vi "Ctor.vi"(8 "error in (no error)":errorcluster) -> (0 "error out":errorcluster, 3 "PanelArray":refnum<class "ArrayManager.lvclass">)   [LabVIEW 2020, in "OOPanel.lvlib" / "ArrayManager.lvclass"]
uses:
  ArrayManager.lvclass
  ArrayPanel/ArrayPanel.lvclass
  UI Refs.ctl
  Events.ctl
  State Ref.ctl
  Event Regs.ctl
  ArrayManager.lvclass/ArrayManager.ctl
  Manager/Manager.lvclass
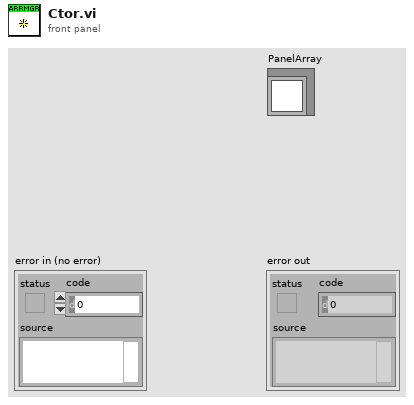
[diagram p1: front panel]
types:
  T1 = typedef "OOPanel.lvlib/ArrayManager.lvclass/Event Regs.ctl" = cluster{"Event Reg":refnum<event-registration>, "Last Update Ticks ms":u32}
  T2 = typedef "OOPanel.lvlib/ArrayManager.lvclass/State Ref.ctl" = cluster{"Running":bool, "Borders":bool, "Total Height":dbl, "Scroll Visible":bool}
  T3 = typedef "OOPanel.lvlib/ArrayManager.lvclass/Events.ctl" = cluster{"Stop":refnum<user-event>, "Update":refnum<user-event>, "Scroll":refnum<user-event>}
  T4 = typedef "OOPanel.lvlib/ArrayManager.lvclass/UI Refs.ctl" = cluster{"SubPanels":refnum<vi>[], "Scrollbar":refnum<vi>, "Panel VI":refnum<vi>, "Container":refnum<vi>}
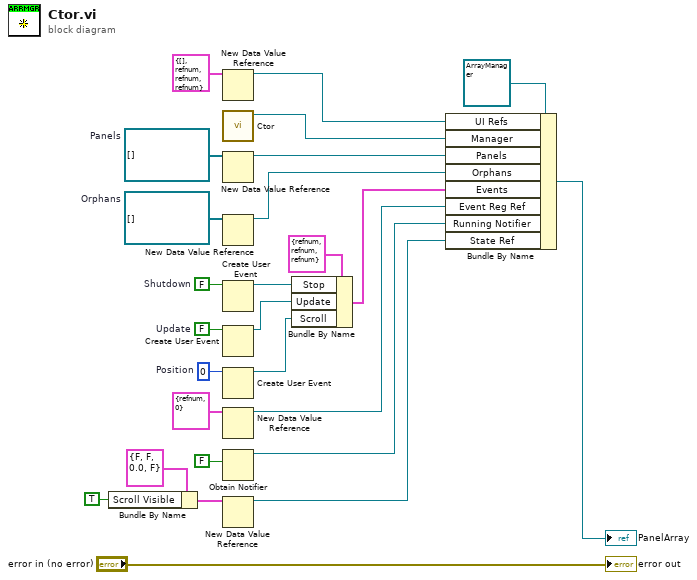
[diagram p0: block diagram]
diagram:
  w5 = 0  # Position
  w13 = FALSE  # Update
  w19 = refnum<class "ArrayPanel.lvclass">[] []  # Orphans
  w20 = refnum<class "ArrayPanel.lvclass">[] []  # Panels
  w22 = FALSE  # Shutdown
  n1 = Bundle By Name(cluster=T2 {"Running"=FALSE, "Borders"=FALSE, "Total Height"=0.0, "Scroll Visible"=FALSE} ("State Ref"), "Scroll Visible"=TRUE) -> (w7:T2)
  n2 = New Data Value Reference(data value=T4 {"SubPanels"=[], "Scrollbar"=refnum, "Panel VI"=refnum, "Container"=refnum} ("UI Refs")) -> (data value reference=w15:refnum<data-value>)  [unwired: 1 in, 1 out]
  n3 = call "Ctor.vi"() -> ("Manager out"=w23:refnum<class "Manager.lvclass">)  [unwired: 10 in, 1 out]
  n4 = New Data Value Reference(data value=w20) -> (data value reference=w18:refnum<data-value>)  [unwired: 1 in, 1 out]
  n5 = New Data Value Reference(data value=w19) -> (data value reference=w17:refnum<data-value>)  [unwired: 1 in, 1 out]
  n6 = Create User Event(user event datatype=w22) -> (user event=w21:refnum<user-event>)  [unwired: 1 in, 1 out]
  n7 = Create User Event(user event datatype=w13) -> (user event=w12:refnum<user-event>)  [unwired: 1 in, 1 out]
  n8 = Create User Event(user event datatype=w5) -> (user event=w4:refnum<user-event>)  [unwired: 1 in, 1 out]
  n9 = New Data Value Reference(data value=T1 {"Event Reg"=refnum, "Last Update Ticks ms"=0} ("Event Reg State")) -> (data value reference=w1:refnum<data-value>)  [unwired: 1 in, 1 out]
  n10 = Obtain Notifier(notification data type=FALSE) -> (notifier out=w10:refnum<notifier>)  [unwired: 3 in, 2 out]
  n11 = New Data Value Reference(data value=w7) -> (data value reference=w8:refnum<data-value>)  [unwired: 1 in, 1 out]
  n12 = Bundle By Name(cluster=T3 {"Stop"=refnum, "Update"=refnum, "Scroll"=refnum} ("Events"), "Stop"=w21, "Update"=w12, "Scroll"=w4) -> (w3:T3)
  n13 = Bundle By Name(cluster=refnum<class "ArrayManager.lvclass"> refnum ("PanelArray in"), "UI Refs"=w15, "Manager"=w23, "Panels"=w18, "Orphans"=w17, "Events"=w3, "Event Reg Ref"=w1, "Running Notifier"=w10, "State Ref"=w8) -> (→"PanelArray":refnum<class "ArrayManager.lvclass">)
  "error out" <- "error in (no error)"
